vi "LV SciSDK FRAME SINGLE.vi"(8 "error in (no error)":errorcluster, 9 "Frame Handle In":T2) -> (0 "error out":errorcluster, 1 "Frame Handle Out":T2, 2 "buffer out":T1, 3 "function return":i32)   [LabVIEW 2021]
uses:
  SciSDK_Labview.lvlib
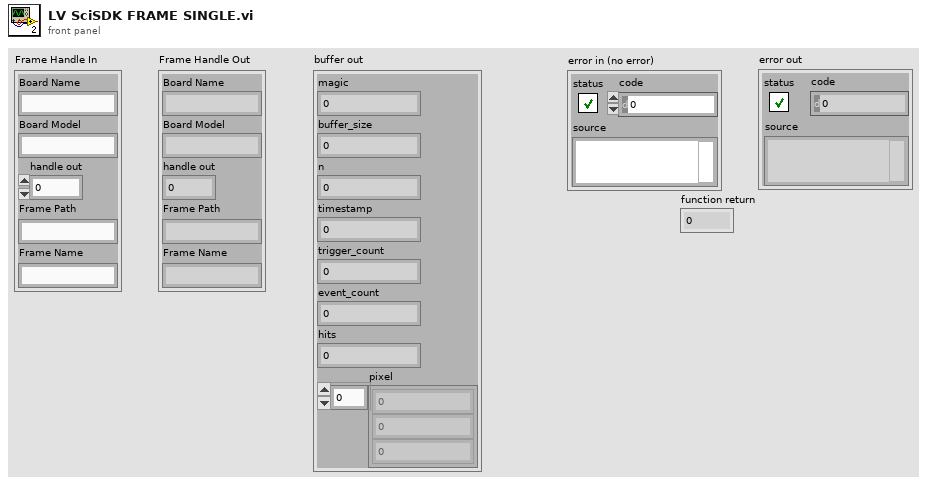
[diagram p1: front panel]
types:
  T1 = cluster{"magic":u32, "buffer_size":u32, "n":u64, "timestamp":u64, "trigger_count":u64, "event_count":u64, "hits":u64, "pixel":u32[]}
  T2 = cluster{"Board Name":string, "Board Model":string, "handle out":u64, "Frame Path":string, "Frame Name":string}
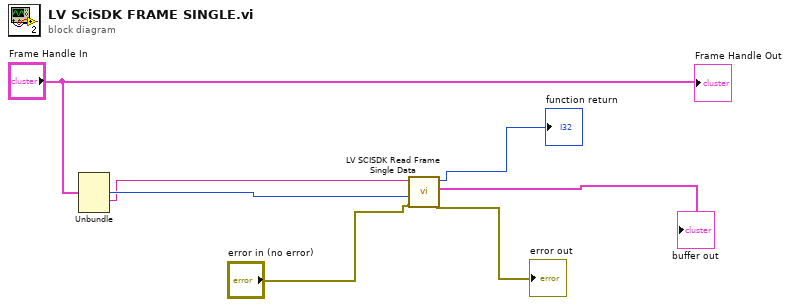
[diagram p0: block diagram]
diagram:
  n1 = Unbundle("Frame Handle In") -> ("handle out"=w3:u64, "Frame Path"=w2:string)  [unwired: 3 out]
  n2 = call "LV SCISDK Read Frame Single Data.vi"("Path"=w2, "handle"=w3, "error in (no error)"="error in (no error)") -> ("function return"=→"function return":i32, "buffer out"=→"buffer out":T1, "error out"=→"error out":errorcluster)  [unwired: 4 in, 1 out]
  "Frame Handle Out" <- "Frame Handle In"
